vi "Aspect Ratio Coral.vi"(11 "Bounds":dbl[](array[numeric])) -> (3 "Score":dbl)   [LabVIEW 2025]
doc: "This VI compares the calculated diameter and convex hull area to compare this shape to a half-hexagon."
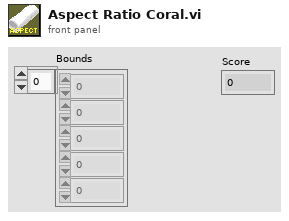
[diagram p1: front panel]
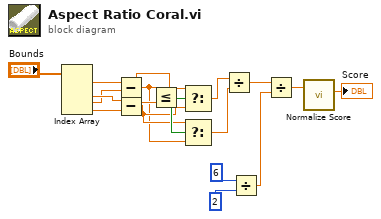
[diagram p0: block diagram]
diagram:
  n1 = Index Array(array="Bounds") -> (element #1=w14:dbl, element #2=w13:dbl, element #3=w12:dbl, element #4=w15:dbl)  [unwired: 4 in]
  n2 = Subtract(x=w14, y=w12) -> (x-y=w2:dbl)
  n3 = Subtract(x=w13, y=w15) -> (x-y=w3:dbl)
  n4 = Less Or Equal?(x=w2, y=w3) -> (x <= y?=w4:bool)
  n5 = Select(t=w2, s=w4, f=w3) -> (s? t:f=w5:dbl)
  n6 = Select(t=w3, s=w4, f=w2) -> (s? t:f=w1:dbl)
  n7 = Divide(x=w5, y=w1) -> (x/y=w11:dbl)
  n8 = Divide(x=6, y=2) -> (x/y=w8:dbl)
  n9 = Divide(x=w11, y=w8) -> (x/y=w7:dbl)
  n10 = call "Normalize Score.vi"("Value"=w7) -> ("Score"=→"Score":dbl)  [unwired: 10 in]
